vi "tlc_Initialize.vi"(7 "Anzahl Kanäle":cluster{"Rows":i32, "Columns":i32}, 8 "error in (no error)":errorcluster, 9 "Consumer Queue Reference.ctl":T2, 10 "Display Queue Reference.ctl":T1, 11 "User Event Reference.ctl":T3) -> (0 "error out":errorcluster)   [LabVIEW 2010]
uses:
  Controls/tlc_User Event Reference.ctl
  Controls/tlc_Consumer Queue Reference.ctl
  Controls/tlc_Consumer Control.ctl
  Controls/tlc_Functions.ctl
  Controls/tlc_Display Queue Reference.ctl
  Controls/tlc_User Interface Command.ctl
  Controls/tlc_User Interface Data Type.ctl
  Modules/Display/tlc_Display_Command Control.ctl
  Modules/Hardware/tlc_Hardware_Command Control.ctl
  Modules/File/tlc_File_Command Control.ctl
  Modules/Cue/tlc_Cue_Information Command.ctl
  Modules/Error/tlc_Error Module Command Control.ctl
  Modules/Error/tlc_Error Module.vi
  Modules/Cue/tlc_Cue Module.vi
  Modules/File/tlc_File Module.vi
  Modules/Hardware/tlc_Hardware Module.vi
  Modules/Display/tlc_Display Module.vi
panel:
  # "Input"
  # "Output"
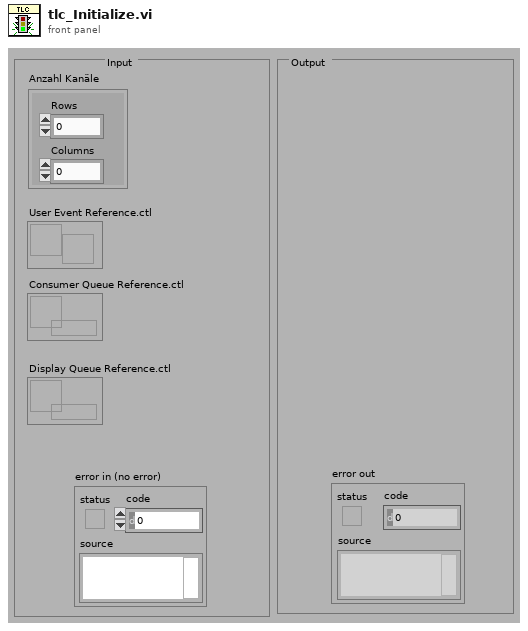
[diagram p1: front panel]
types:
  T1 = typedef "tlc_Display Queue Reference.ctl" = refnum<queue>
  T2 = typedef "tlc_Consumer Queue Reference.ctl" = refnum<queue>
  T3 = typedef "tlc_User Event Reference.ctl" = refnum<user-event>
  T4 = typedef "tlc_User Interface Data Type.ctl" = enum16{"Initialize", "Initialize Front Panel", "Update Front Panel Channels", "Select Cue in Cue List", "Enable/Disable Front Panel Controls", "Update Cue List", "Stop"}
  T5 = typedef "tlc_Display_Command Control.ctl" = enum16{"Initialize", "Update UI", "Shutdown"}
  T6 = typedef "tlc_Hardware_Command Control.ctl" = enum16{"Initialize", "Write", "Shutdown"}
  T7 = typedef "tlc_File_Command Control.ctl" = enum16{"Init", "Speicher Lichtersets", "Lade Lichtersets", "Ende"}
  T8 = typedef "tlc_Cue_Information Command.ctl" = enum16{"Add Lichtset", "Get Lichtset Werte", "Set Lichtset Werte", "Get Anzahl Lichtersets", "Init", "Get Leeres Lichterset"}
  T9 = typedef "tlc_Error Module Command Control.ctl" = enum16{"Initialize", "Handle Errors", "Report Errors"}
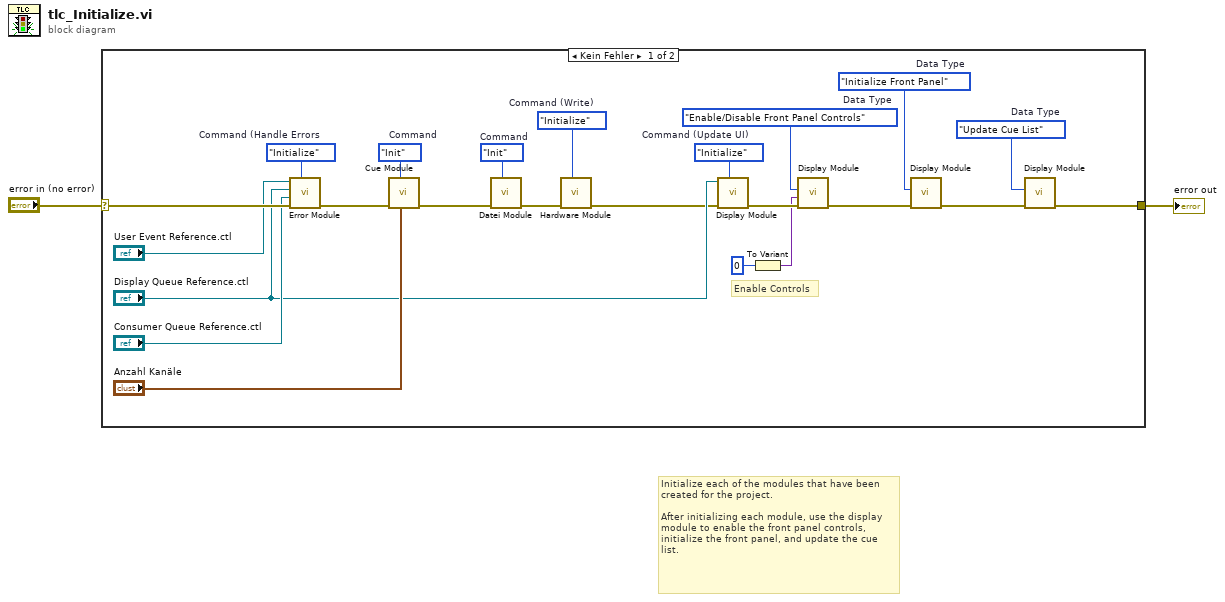
[diagram p0: block diagram]
diagram:
  # "Initialize each of the modules that have been created for the project.\n\nAfter initializing each module, use the display module to enable the front panel controls, initialize the front panel, and update the cue list."
  n1 = case shown="Kein Fehler" "error in (no error)" {
    selector: "error in (no error)" -> [w25 w26]
    tunnel: [w22 w26] -> w1
    frame No Error {
      w6 = tlc_User_Interface_Data_Type."Update Cue List"  # Data Type
      w7 = tlc_User_Interface_Data_Type."Initialize Front Panel"  # Data Type
      w8 = tlc_User_Interface_Data_Type."Enable/Disable Front Panel Controls"  # Data Type
      w9 = tlc_Display_Command_Control."Initialize"  # Command (Update UI)
      w10 = tlc_Hardware_Command_Control."Initialize"  # Command (Write)
      w11 = tlc_File_Command_Control."Init"  # Command
      w12 = tlc_Cue_Information_Command."Init"  # Command
      w13 = tlc_Error_Module_Command_Control."Initialize"  # Command (Handle Errors
      # "Enable Controls"
      n2 = call "Error Module.vi"("Command (Handle Errors)"=w13, "error in (no error)"=w25, "tlc_Consumer Queue Reference.ctl"="Consumer Queue Reference.ctl", "tlc_Display Queue Reference.ctl"="Display Queue Reference.ctl", "tlc_User Event Reference.ctl"="User Event Reference.ctl") -> ("error out"=w17:errorcluster)  [unwired: 5 in, 1 out]
      n3 = call "Cue Module.vi"("Number of Channels"="Anzahl Kanäle", "Command"=w12, "error in (no error)"=w17) -> ("error out"=w16:errorcluster)  [unwired: 5 in, 2 out]
      n4 = call "Datei Module.vi"("Command"=w11, "error in (no error)"=w16) -> ("error out"=w3:errorcluster)  [unwired: 8 in, 1 out]
      n5 = call "Hardware Module.vi"("Command (Write)"=w10, "error in (no error)"=w3) -> ("error out"=w15:errorcluster)  [unwired: 9 in]
      n6 = call "Display Module.vi"("Command (Update UI)"=w9, "error in (no error)"=w15, "tlc_Display Queue Reference.ctl"="Display Queue Reference.ctl") -> ("error out"=w14:errorcluster)  [unwired: 8 in]
      n7 = To Variant(anything=u8 0) -> (Variant=w5:variant)
      n8 = call "Display Module.vi"("error in (no error)"=w14, "Data"=w5, "Data Type"=w8) -> ("error out"=w24:errorcluster)  [unwired: 8 in]
      n9 = call "Display Module.vi"("error in (no error)"=w24, "Data Type"=w7) -> ("error out"=w23:errorcluster)  [unwired: 9 in]
      n10 = call "Display Module.vi"("error in (no error)"=w23, "Data Type"=w6) -> ("error out"=w22:errorcluster)  [unwired: 9 in]
    }
    frame Error {
    }
  }
  "error out" <- w1
